vi "20170516-lecture4-2 prof Login.vi"() -> (2 "Correct":bool)   [LabVIEW 2014]
panel:
  in  "stop":bool
  in  "Password":string
  in  "Username":string
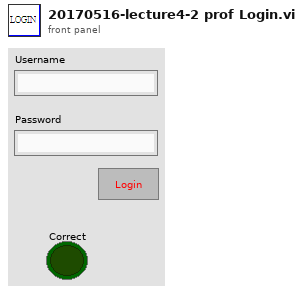
[diagram p1: front panel]
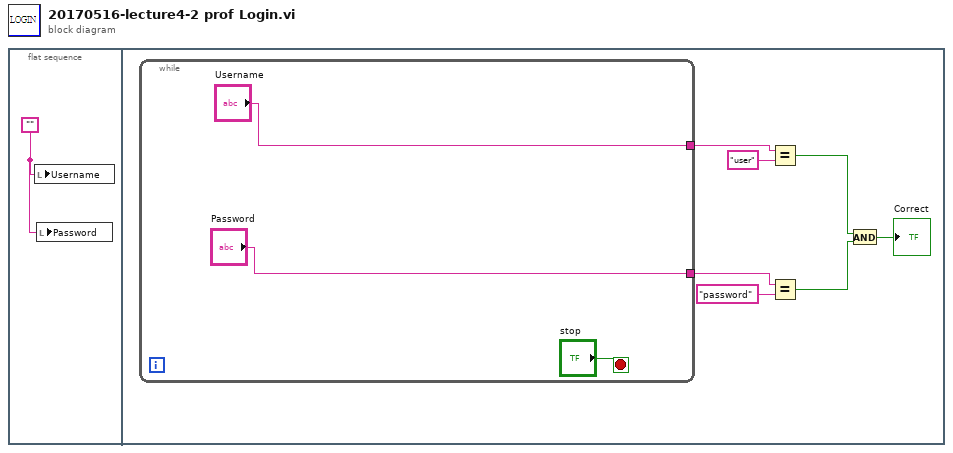
[diagram p0: block diagram]
diagram:
  n1 = flat-sequence {
    frame #0 {
      w1 = ""
      n2 = local write "Username"(w1) -> ()
      n3 = local write "Password"(w1) -> ()
    }
    frame #1 {
      n4 = while {
        tunnel: ["Username"] -> w3
        tunnel: ["Password"] -> w2
        stop <- "stop" stop-if-true
      }
      n5 = Equal?(x=w3, y="user") -> (x = y?=w6:bool)
      n6 = Equal?(x=w2, y="password") -> (x = y?=w7:bool)
      n7 = And(x=w6, y=w7) -> (x .and. y?=→"Correct":bool)
    }
  }
